vi "Initialization VI.vi"(8 "error in (no error)":errorcluster, 10 "Custom XML":string, 11 "Device Item Ref in":T1 format="%.0x") -> (0 "error out":errorcluster, 3 "Device Item Ref out":T1 format="%.0x")   [LabVIEW 2020, in "Profile Interpolation System Explorer.lvlib"]
uses:
  Profile Interpolation System Explorer.lvlib
  <vilib>/NI VeriStand/Custom Device API/Custom Device Item Ref.ctl
  Shared/Types/FG Action.ctl
  Shared/Types/Interpolation Settings.ctl
  Shared/SubVIs/Constants.vi
  <vilib>/NI VeriStand/Custom Device API/NI VeriStand - Get Item Property.vi
  <vilib>/NI VeriStand/Custom Device API/Get Item Property (Path).vi
  <vilib>/NI VeriStand/Custom Device API/Get Item Property (Boolean).vi
  <vilib>/NI VeriStand/Custom Device API/NI VeriStand - Set Item Property.vi
  <vilib>/NI VeriStand/Custom Device API/Set Item Property (Path).vi
  <vilib>/NI VeriStand/Custom Device API/Set Item Property (Boolean).vi
  <vilib>/NI/NI VeriStand Custom Device Import and Export Tool/ImportExport.lvlib
  Shared/Profile Interpolation Shared.lvlib
  <vilib>/NI VeriStand/Custom Device API/Custom Device API.lvlib
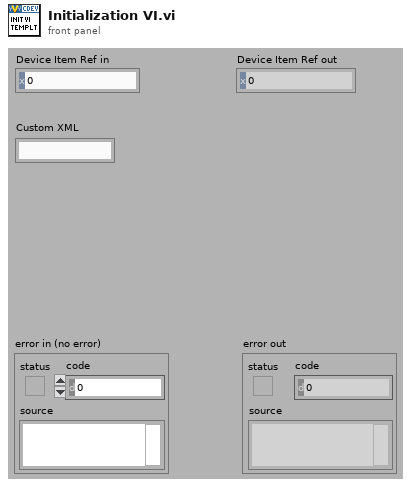
[diagram p1: front panel]
types:
  T1 = typedef "Custom Device API.lvlib/Custom Device Item Ref.ctl" = u64
  T2 = typedef "Profile Interpolation Shared.lvlib/Interpolation Settings.ctl" = cluster{"Interpolation File":path, "Create Limit Channels?":bool}
  T3 = typedef "Profile Interpolation Shared.lvlib/FG Action.ctl" = enum8{"GET", "SET"}
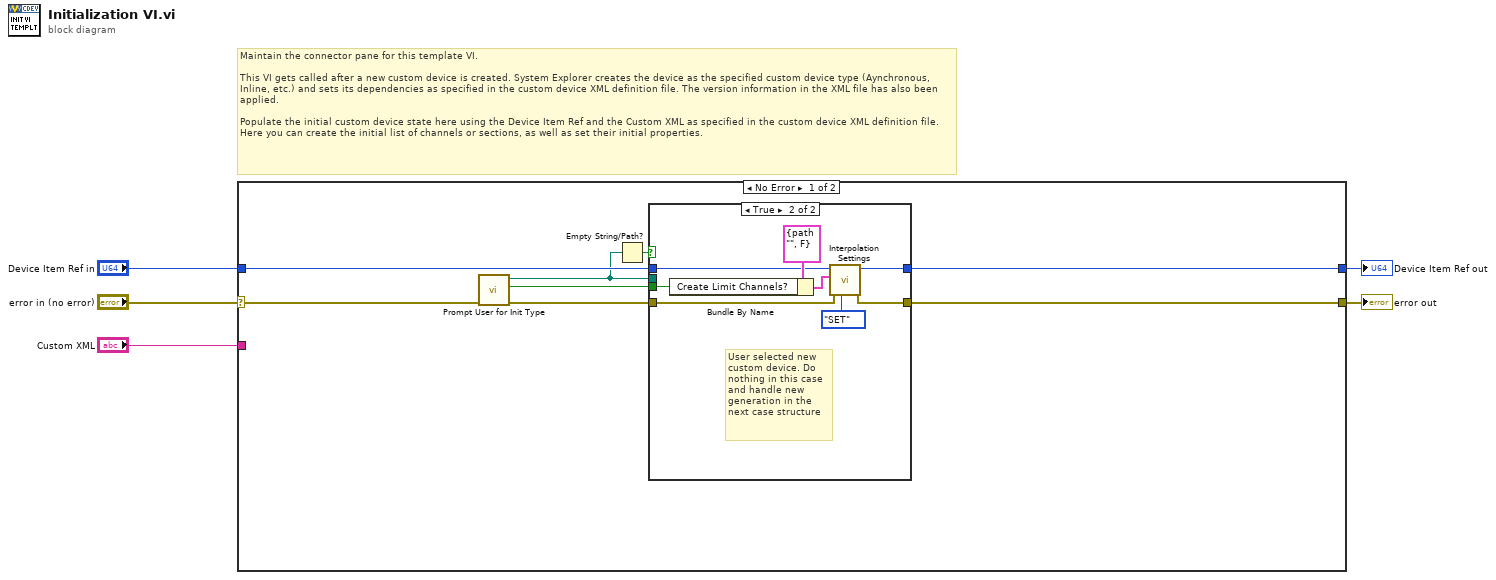
[diagram p0: block diagram]
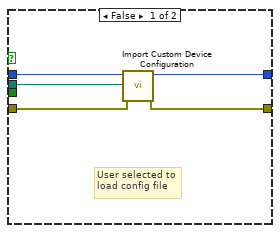
[diagram p2: hidden frame]
diagram:
  # "Maintain the connector pane for this template VI.\n\nThis VI gets called after a new custom device is created. System Explorer creates the device as the specified custom device type (Aynchronous, Inline, etc.) and sets its dependencies as specified in the custom device XML definition file. The version information in the XML file has also been applied.\n\nPopulate the initial custom device state here using the Device Item Ref and the Custom XML as specified in the custom device XML definition file. Here you can create the initial list of channels or sections, as well as set their initial properties."
  n1 = case shown="No Error" "error in (no error)" {
    selector: "error in (no error)" -> [w12 w28]
    tunnel: [w6 w28] -> w5
    tunnel: [w7 w27] -> w3
    tunnel: "Device Item Ref in" -> [w13 w27]
    tunnel: "Custom XML" -> [_ _]
    frame No Error {
      n2 = call "Prompt User for Init Type.vi"("error in (no error)"=w12) -> ("error out"=w11:errorcluster, "Create Limit Channels? out"=w8:bool, "Path out"=w9:path)  [unwired: 8 in]
      n3 = Empty String/Path?(string/path=w9) -> (empty?=w10:bool)
      n4 = case shown="True" w10 {
        tunnel: w13 -> [w18 w22]
        tunnel: [w17 w21] -> w7
        tunnel: w11 -> [w16 w25]
        tunnel: [w15 w24] -> w6
        tunnel: w9 -> [w14 _]
        tunnel: w8 -> [_ w20]
        frame False {
          # "User selected to\nload config file"
          n5 = call <vilib>:"Import Custom Device Configuration.vi"("error in (no error)"=w16, "Path"=w14, "NodeID"=w18) -> ("error out"=w15:errorcluster, "NodeID out"=w17:u64)  [unwired: 6 in, 1 out]
        }
        frame True {
          # "User selected new\ncustom device. Do\nnothing in this case\nand handle new\ngeneration in the\nnext case structure"
          n6 = Bundle By Name(cluster=T2 {"Interpolation File"=path "", "Create Limit Channels?"=FALSE} ("Interpolation Settings"), "Create Limit Channels?"=w20) -> (w19:T2)
          n7 = call "Interpolation Settings.vi"("Action"=FG_Action."SET", "error in (no error)"=w25, "Interpolation Settings"=w19, "Item Ref"=w22) -> ("error out"=w24:errorcluster, "Item Ref out"=w21:T1)  [unwired: 5 in, 1 out]
        }
      }
    }
    frame Error {
    }
  }
  "error out" <- w5
  "Device Item Ref out" <- w3
